vi "setAUX.vi"(8 "error in (no error)":errorcluster, 9 "AUX (V)":dbl, 10 "Channel":i32=1 min=1 max=16, 11 "Instrument.LockinAPI in":refnum<class "Instrument.LockinAPI.lvclass">) -> (0 "error out":errorcluster, 3 "Instrument.LockinAPI out":refnum<class "Instrument.LockinAPI.lvclass">)   [LabVIEW 2019, in "Instrument.LockinAPI.lvclass"]
doc: "API to configure an AO DC offset.\n\nSpecify which channel you want to change and the value you want to set.\n\nIf address=\"\", this API reads from localhost\nIf address is remote lockin, you need to add this computer to allowed whitelist on the lockin computer you are trying to access."
uses:
  Instrument.LockinAPI.lvclass
  C:/Users/patrick/Documents/GitHub/Instrument-Framework/lvsrc/Instrument/Instrument.lvclass
  Typedefs/API/LockinAPI.Commands--Enum.ctl
  Typedefs/API/LockinAPI.setAUX--cluster.ctl
  03b2bfdc-50cd-46c3-b599-93f9cb353570.vi
  03b2bfdc-50cd-46c3-b599-93f9cb353570.vi/435308b9-5942-46b6-874d-525fcd91f5b1.vi
  03b2bfdc-50cd-46c3-b599-93f9cb353570.vi/435308b9-5942-46b6-874d-525fcd91f5b1.vi/03a159f0-872f-48f3-a0d1-f404c20d438a.vi
  03b2bfdc-50cd-46c3-b599-93f9cb353570.vi/435308b9-5942-46b6-874d-525fcd91f5b1.vi/f4ff504f-ac32-429e-9f6f-cdfa3b066111.vi
  03b2bfdc-50cd-46c3-b599-93f9cb353570.vi/435308b9-5942-46b6-874d-525fcd91f5b1.vi/037e8f0d-866c-4fdd-a2ce-98957b1ad5a5.vi
  <vilib>/JDP Science/JSONtext/Make JSON Array.vi
  03b2bfdc-50cd-46c3-b599-93f9cb353570.vi/435308b9-5942-46b6-874d-525fcd91f5b1.vi/f4ff504f-ac32-429e-9f6f-cdfa3b066111.vi/c5284adb-5d16-4c14-a592-b8b8be9dacb5.vi
  03b2bfdc-50cd-46c3-b599-93f9cb353570.vi/435308b9-5942-46b6-874d-525fcd91f5b1.vi/037e8f0d-866c-4fdd-a2ce-98957b1ad5a5.vi/73e09e33-d270-4172-ae0f-c4da78ff9325.vi
  03b2bfdc-50cd-46c3-b599-93f9cb353570.vi/435308b9-5942-46b6-874d-525fcd91f5b1.vi/037e8f0d-866c-4fdd-a2ce-98957b1ad5a5.vi/927bafea-0fe7-49ca-b25a-16679e8ba8c1.vi
  Instrument/API/Enum to String.vi
  Instrument/Private/Get RC Connection Status.vi
  <vilib>/JDP Science/JSONtext/Variant to JSON Text.vi
  <vilib>/JDP Science/JSONtext/support/Format JSON Array Text.vi
  Instrument/API/Send and Receive.vi
  <vilib>/JDP Science/JSONtext/JSON text to Variant.vi
  <vilib>/Utility/Data Type/Get Type Information.vi
  <vilib>/JDP Science/JSONtext/LVClass Serializer/JSONtext LVClass Serializer.lvclass
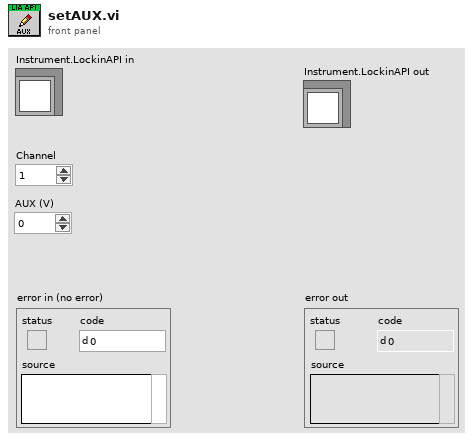
[diagram p1: front panel]
types:
  T1 = typedef "Instrument.LockinAPI.lvclass/LockinAPI.setAUX--cluster.ctl" = cluster{"AO Channel":i32, "AUX (V)":dbl}
  T2 = typedef "Instrument.LockinAPI.lvclass/LockinAPI.Commands--Enum.ctl" = enum16{"setAI", "setAO", "setAO_Amplitude", "setAO_DC", "setAO_Frequency", "setAO_Phase", "setAO_Function", "setAO_I+", "setREF", "setREF_Frequency", "setREF_Phase", "setREF_TC", "setREF_Roll-Off", "setDAQ", "setSampling", "setOffset", "setState", "getState", "getAO", "getAI", "getResults", "getSampling", "getAOconfig", "getREFconfig", "setInputGain", "setOutputGain", "getInputGain", "getOutputGain", "setSamplingMode", "getSamplingMode", "setSweep", "setSweepTime", "setSweepTable", "getStatus", "getSweepResults", "getSweepWaveforms", "startSweep", "stopSweep", "setAUX", "getAUX"}
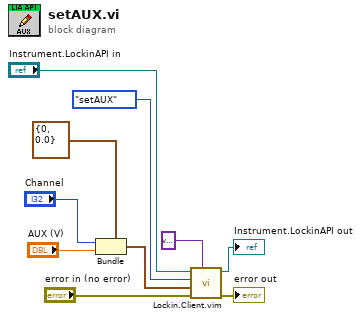
[diagram p0: block diagram]
diagram:
  n1 = Bundle(cluster=T1 {"AO Channel"=0, "AUX (V)"=0.0} ("setAUX"), "AO Channel"="Channel", "AUX (V)"="AUX (V)") -> (w10:T1)
  n2 = call "Lockin.Client.vim"("Data Out type"=variant, "error in (no error)"="error in (no error)", "Data"=w10, "Command"=LockinAPI.Commands--Enum."setAUX", "Instrument.LockinAPI in"="Instrument.LockinAPI in") -> ("error out"=→"error out":errorcluster, "Instrument.LockinAPI out"=→"Instrument.LockinAPI out":refnum<class "Instrument.LockinAPI.lvclass">)  [unwired: 4 in, 1 out]
